vi "Angle Chooser.vi"(5 "Forearm Angle Initial":dbl, 7 "Backarm Angle Initial":dbl, 8 "Forearm Angle 2":dbl, 9 "Backarm Angle 2":dbl, 10 "Forearm Angle 1":dbl, 11 "Backarm Angle 1":dbl) -> (2 "final Forearm Angle":dbl, 3 "final Backarm Angle":dbl)   [LabVIEW 2017]
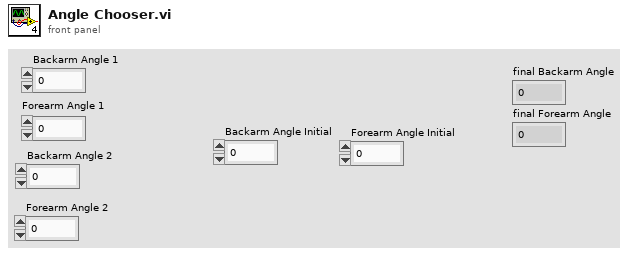
[diagram p1: front panel]
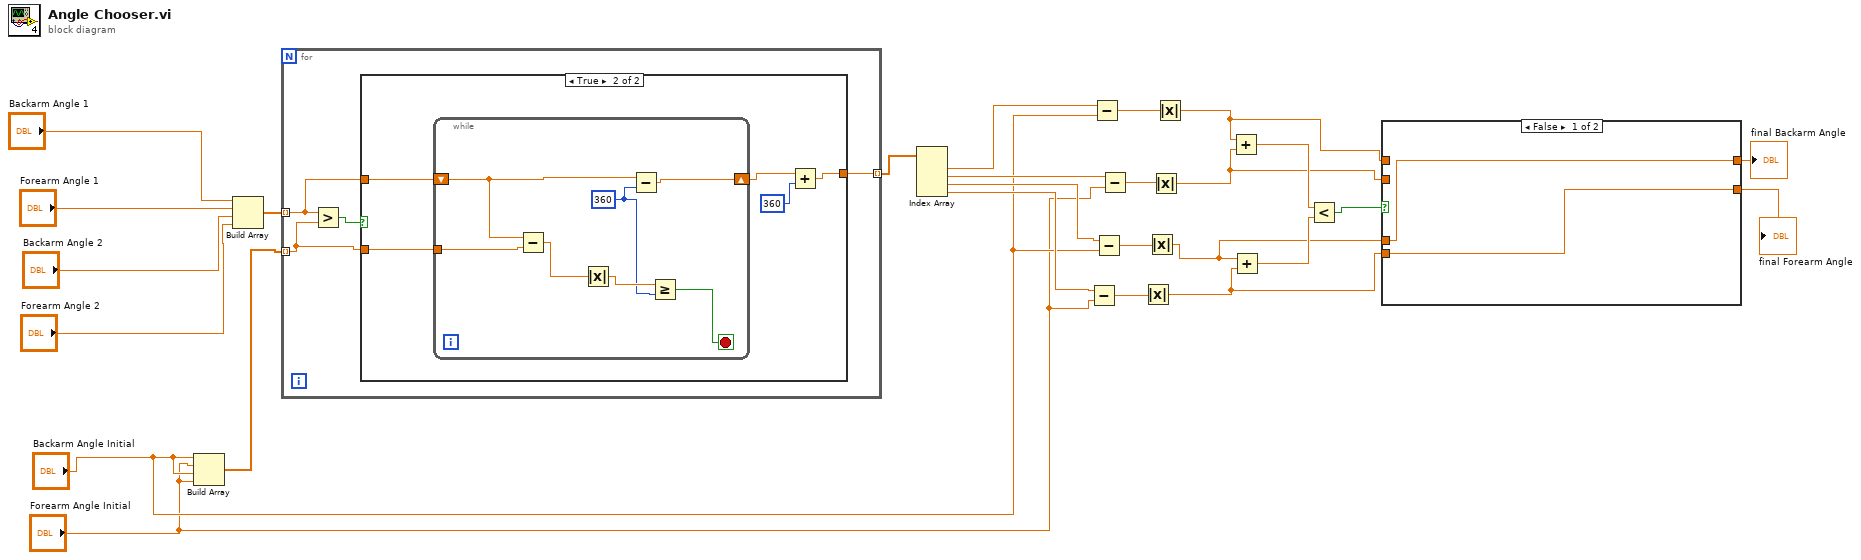
[diagram p0: block diagram]
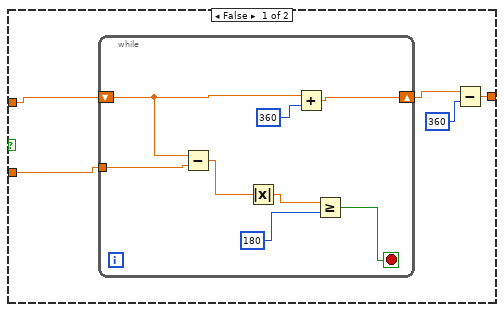
[diagram p2: hidden frame]
diagram:
  n1 = Build Array("Backarm Angle Initial", "Forearm Angle Initial", "Backarm Angle Initial", "Forearm Angle Initial") -> (w8:dbl[])
  n2 = Build Array("Backarm Angle 1", "Forearm Angle 1", "Backarm Angle 2", "Forearm Angle 2") -> (w9:dbl[])
  n3 = for {
    tunnel: w9 -> [w29] mode=indexing
    tunnel: w8 -> [w28] mode=indexing
    tunnel: [w27] -> w7 mode=indexing
    n4 = Greater?(x=w29, y=w28) -> (0:w30:bool)
    n5 = case shown="True" w30 {
      tunnel: w29 -> [w33 w48]
      tunnel: w28 -> [w32 w47]
      tunnel: [w31 w44] -> w27
      frame False {
        n6 = while {
          shift-right: [w43] -> w35
          shift-left: w33 -> [w42]
          tunnel: w32 -> [w41]
          stop <- w38 stop-if-true
          n7 = Subtract(x=w42, y=w41) -> (x-y=w40:dbl)
          n8 = Absolute Value(x=w40) -> (abs(x)=w39:dbl)
          n9 = Add(x=w42, y=360) -> (x+y=w43:dbl)
          n10 = Greater Or Equal?(x=w39, y=180) -> (x >= y?=w38:bool)
        }
        n11 = Subtract(x=w35, y=360) -> (x-y=w31:dbl)
      }
      frame True {
        n12 = while {
          shift-right: [w55] -> w46
          shift-left: w48 -> [w54]
          tunnel: w47 -> [w53]
          stop <- w50 stop-if-true
          w49 = 360
          n13 = Subtract(x=w54, y=w53) -> (x-y=w52:dbl)
          n14 = Absolute Value(x=w52) -> (abs(x)=w51:dbl)
          n15 = Subtract(x=w54, y=w49) -> (x-y=w55:dbl)
          n16 = Greater Or Equal?(x=w51, y=w49) -> (x >= y?=w50:bool)
        }
        n17 = Add(x=w46, y=360) -> (x+y=w44:dbl)
      }
    }
  }
  n18 = Index Array(array=w7) -> (element #1=w6:dbl, element #2=w5:dbl, element #3=w4:dbl, element #4=w3:dbl)  [unwired: 4 in]
  n19 = Subtract(x=w3, y="Forearm Angle Initial") -> (x-y=w23:dbl)
  n20 = Subtract(x=w6, y="Backarm Angle Initial") -> (x-y=w26:dbl)
  n21 = Subtract(x=w4, y="Backarm Angle Initial") -> (x-y=w24:dbl)
  n22 = Subtract(x=w5, y="Forearm Angle Initial") -> (x-y=w25:dbl)
  n23 = Absolute Value(x=w23) -> (abs(x)=w16:dbl)
  n24 = Absolute Value(x=w24) -> (abs(x)=w17:dbl)
  n25 = Absolute Value(x=w25) -> (abs(x)=w18:dbl)
  n26 = Absolute Value(x=w26) -> (abs(x)=w19:dbl)
  n27 = Add(x=w19, y=w18) -> (x+y=w21:dbl)
  n28 = Add(x=w17, y=w16) -> (x+y=w20:dbl)
  n29 = Less?(x=w21, y=w20) -> (x < y?=w22:bool)
  n30 = case shown="False" w22 {
    tunnel: w19 -> [_ w59]
    tunnel: w18 -> [_ w58]
    tunnel: [w57 w59] -> w15
    tunnel: [w56 w58] -> w14
    tunnel: w17 -> [w57 _]
    tunnel: w16 -> [w56 _]
    frame False {
    }
    frame True {
    }
  }
  "final Backarm Angle" <- w15
  "final Forearm Angle" <- w14
